vi "API - On Demand - Write 1 Digital Output Sample on Demand.vi"(8 "error in":errorcluster, 9 "Boolean Data In":bool=TRUE, 10 "Digital Output Channel Number":i32, 11 "DAQiFi Device Properties In":T1) -> (0 "error out":errorcluster, 3 "DAQiFi Device Properties Out":T1)   [LabVIEW 2021]
doc: "Write a single digital output value to the DAQ\n-Enable channel\n-Set state of digital output"
uses:
  TypeDefs/TypeDef - Cluster of DAQiFi Device Properties.ctl
  TypeDefs/Enum - Connection Type.ctl
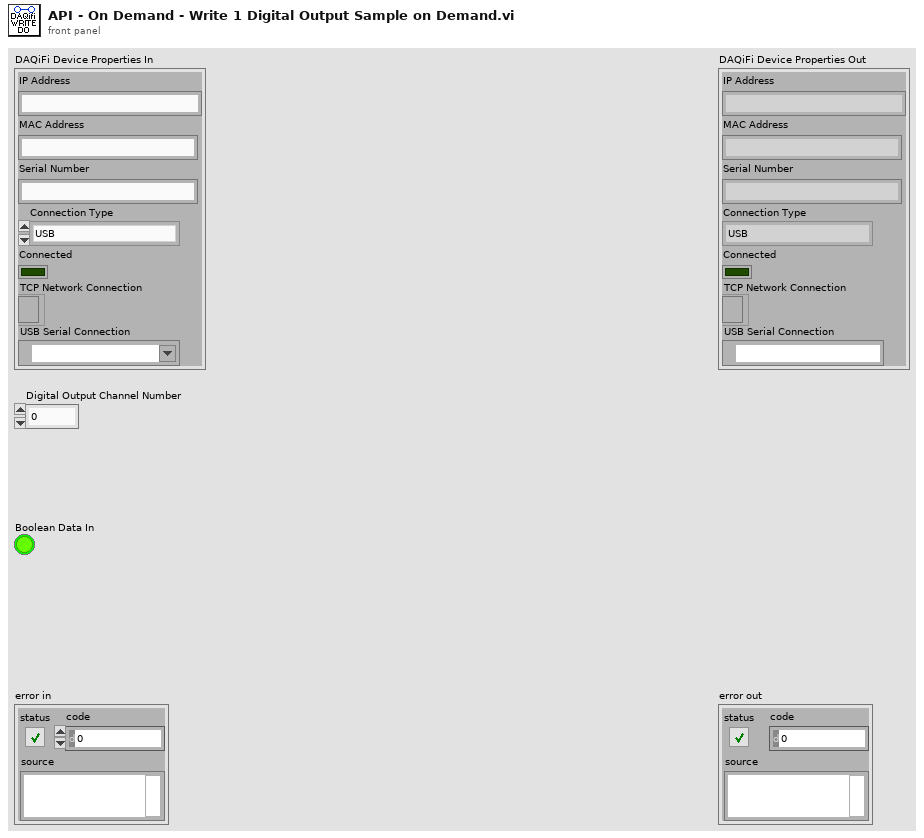
[diagram p1: front panel]
types:
  T1 = typedef "TypeDef - Cluster of DAQiFi Device Properties.ctl" = cluster{"IP Address":string, "MAC Address":string, "Serial Number":string, "Connection Type":T2, "Connected":bool, "TCP Network Connection":refnum<k5>, "USB Serial Connection":refnum<visa-resource-name>}
  T2 = typedef "Enum - Connection Type.ctl" = enum16{"USB", "TCP"}
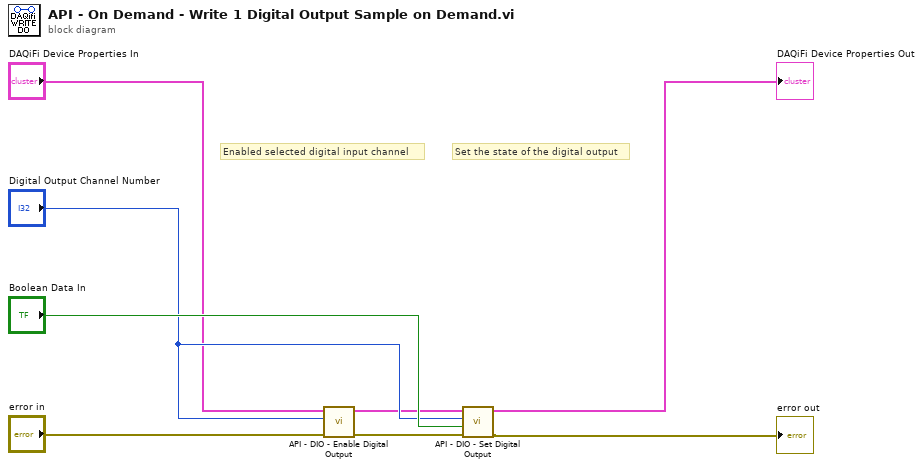
[diagram p0: block diagram]
diagram:
  # "Set the state of the digital output"
  # "Enabled selected digital input channel"
  n1 = call "API - DIO - Enable Digital Output.vi"("error in"="error in", "Channel Number"="Digital Output Channel Number", "DAQiFi Device Properties In"="DAQiFi Device Properties In") -> ("error out"=w7:errorcluster, "DAQiFi Device Properties Out"=w3:T1)  [unwired: 7 in]
  n2 = call "API - DIO - Set Digital Output.vi"("error in"=w7, "State"="Boolean Data In", "Channel Number"="Digital Output Channel Number", "DAQiFi Device Properties In"=w3) -> ("error out"=→"error out":errorcluster, "DAQiFi Device Properties Out"=→"DAQiFi Device Properties Out":T1)  [unwired: 6 in]
